vi "New from Source (Factory).vi"(6 "Branch (Default)":string, 7 "Logger":refnum<class "Logger.lvclass">, 8 "error in (no error)":errorcluster, 9 "Folder":path, 10 "Source":string, 11 "Type":string) -> (0 "error out":errorcluster, 3 "PackageAbstract out":refnum<class "PackageAbstract.lvclass">)   [LabVIEW 2020, in "GPack.lvlib" / "PackageAbstract.lvclass"]
uses:
  PackageAbstract.lvclass
  Logger/Logger.lvclass
  GPack.lvlib
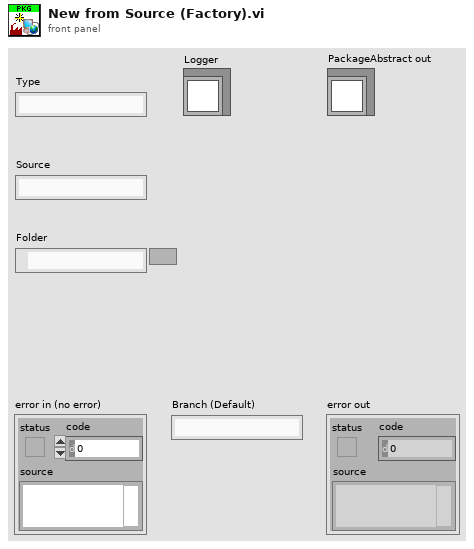
[diagram p1: front panel]
types:
  T1 = typedef "GPack.lvlib/Package Info.ctl" = cluster{"Name":string, "Type":string, "Host":string, "Path":string, "Branch":string, "Version":string, "License":string}
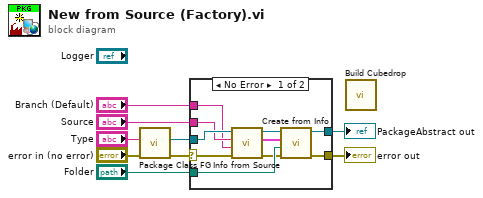
[diagram p0: block diagram]
diagram:
  n1 = call "Package Class FG.vi"("error in (no error)"="error in (no error)", "Package Type (All)"="Type") -> ("error out"=w8:errorcluster, "Package Class"=w7:refnum<class "PackageAbstract.lvclass">)  [unwired: 7 in, 1 out]
  n2 = case shown="No Error" w8 {
    selector: w8 -> [w19 w20]
    tunnel: w7 -> [w14 _]
    tunnel: [w18 w20] -> w6
    tunnel: [w17 _] -> w5
    tunnel: "Folder" -> [w16 _]
    tunnel: "Source" -> [w12 _]
    tunnel: "Branch (Default)" -> [w11 _]
    frame No Error {
      n3 = call-dynamic "Info from Source.vi"("error in (no error)"=w19, "Branch (Default)"=w11, "Source"=w12, "Package in"=w14) -> ("error out"=w15:errorcluster, "Package Info"=w10:T1, "Package out"=w13:refnum<class "PackageAbstract.lvclass">)  [unwired: 4 in, 1 out]
      n4 = call-dynamic "Create from Info.vi"("error in (no error)"=w15, "Folder"=w16, "Package Info"=w10, "Package in"=w13) -> ("error out"=w18:errorcluster, "Package out"=w17:refnum<class "PackageAbstract.lvclass">)  [unwired: 6 in]
    }
    frame Error {
    }
  }
  "error out" <- w6
  "PackageAbstract out" <- w5
  n5 = call "Build Cubedrop.vi"() -> ()  [unwired: 12 in]
